vi "Track_Showing.vi"(3 "NewNodeM":cluster{"NewNodeM[0]":dbl, "NewNodeM[1]":dbl}, 5 "Image In 2":T1, 7 "数值":dbl) -> (6 "Image Out 2":T1)   [LabVIEW 2014]
doc: "在二维图中显示小助手的实时位置"
uses:
  <vilib>/vision/Image Controls.llb/IMAQ Image.ctl
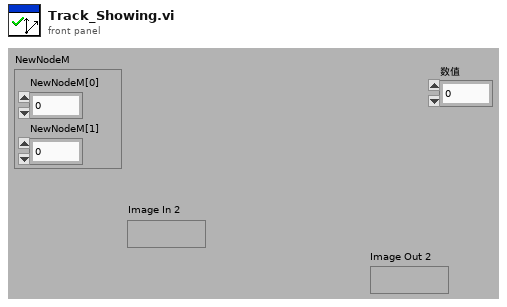
[diagram p1: front panel]
types:
  T1 = typedef "IMAQ Image.ctl" = refnum<image>
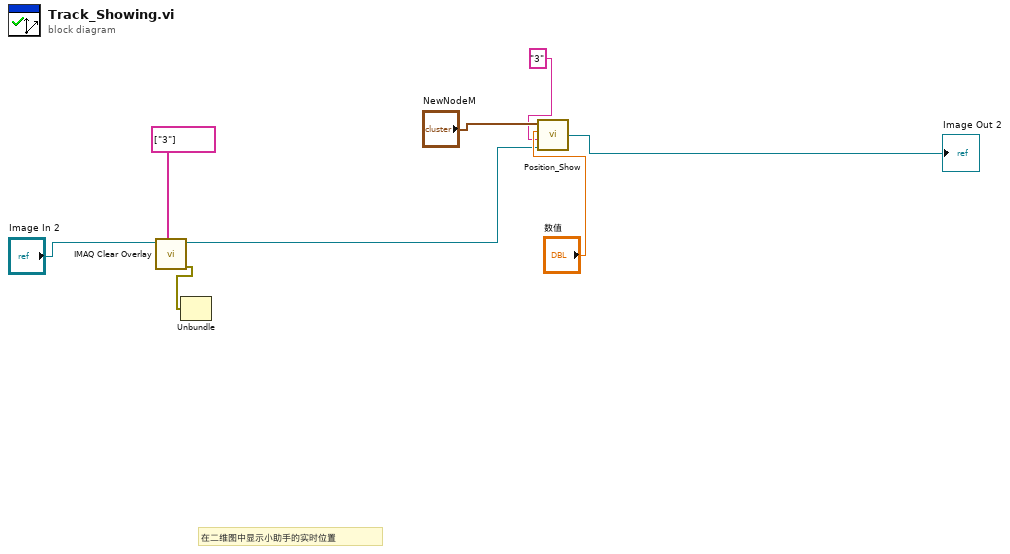
[diagram p0: block diagram]
diagram:
  # "在二维图中显示小助手的实时位置"
  n1 = call "IMAQ Clear Overlay"("Groups"=string[] ["3"], "Image"="Image In 2") -> ("error out"=w7:errorcluster, "Image Out"=w2:T1)  [unwired: 8 in]
  n2 = Unbundle(w7) -> ()  [unwired: 3 out]
  n3 = call "Position_Show.vi"("Image Out 4"=w2, "Group 2"="3" ("Group"), "数值"="数值", "NewNodeM 2"="NewNodeM") -> ("Image Out 3"=→"Image Out 2":T1)  [unwired: 2 in]
